vi "ge_PreviewWfm.vi"(6 "Rate Class":T1, 7 "ChassisCfg":refnum<class "ChassisCfg.lvclass">, 8 "error in":errorcluster, 10 "Chassis Name":string, 11 "Selected Group":refnum<class "ChanGrp.lvclass">) -> (0 "error out":errorcluster)   [LabVIEW 2012]
uses:
  Classes/Cfg Grandmaster/Class Chan Group/ChanGrp.lvclass
  Classes/Cfg Grandmaster/Class Chassis Cfg/ChassisCfg.lvclass
  Common/Controls/TE_Designator.ctl
  <vilib>/Utility/miscctls.llb/LVRowAndColumnTypeDef.ctl
  Classes/Cfg Grandmaster/Class Chan Group/Read GroupChans.vi
  Classes/Cfg Grandmaster/Class Chan Group/Read GrpName.vi
  Classes/Cfg Grandmaster/Class Chan Group/Read MeasType.vi
  Classes/Cfg Grandmaster/Class Timing Group/Read Rate.vi
  Classes/Measurements/Class Channel/Read ChanName.vi
  Classes/Measurements/Class Channel/Read Alias.vi
  Classes/Measurements/Class Channel/Channel.lvclass
  Classes/Cfg Grandmaster/Class Timing Group/TimingGrp.lvclass
panel:
  in  "Legend LB":i32[](listbox)
  out "Wfm Graph":waveform(sgl)[](graph)
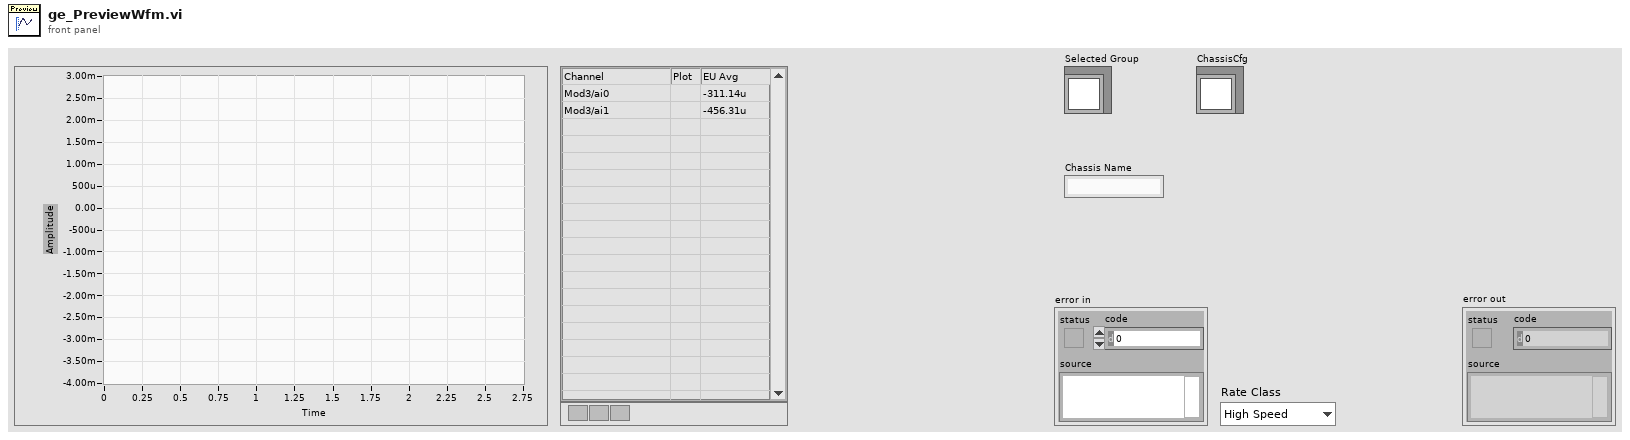
[diagram p1: front panel]
types:
  T1 = typedef "TE_Designator.ctl" = enum16{"High Speed", "Low Speed"}
  T2 = typedef "ge_MeasType.ctl" = enum16{"Voltage", "Frequency", "Tachometer", "Dynamic", "Thermocouple", "RTD", "Strain", "Current", "Resistance"}
  T3 = typedef "LVRowAndColumnTypeDef.ctl" = cluster{"Row":i32, "Column":i32}
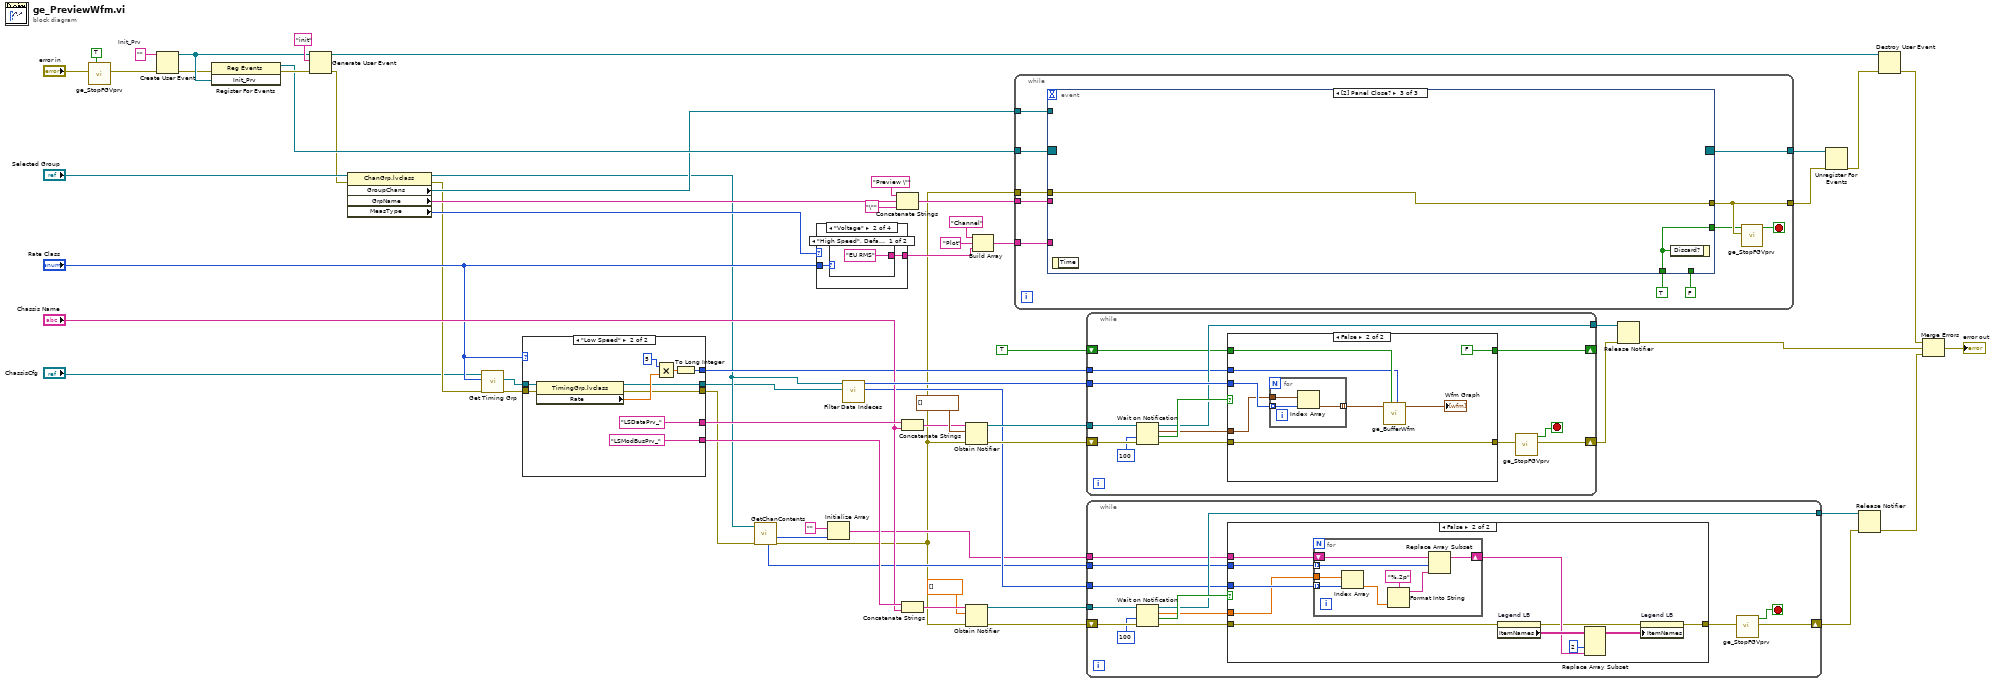
[diagram p0: block diagram]
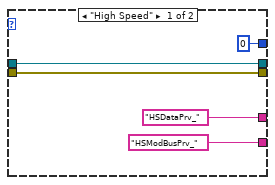
[diagram p2: hidden frame]
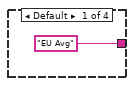
[diagram p3: hidden frame]
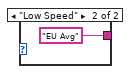
[diagram p4: hidden frame]
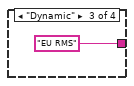
[diagram p5: hidden frame]
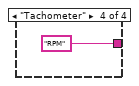
[diagram p6: hidden frame]
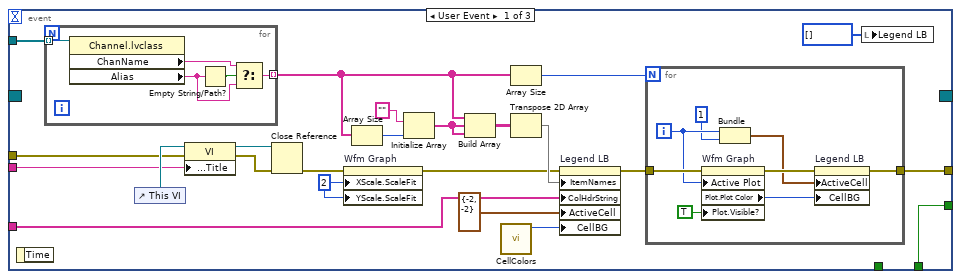
[diagram p8: hidden frame]
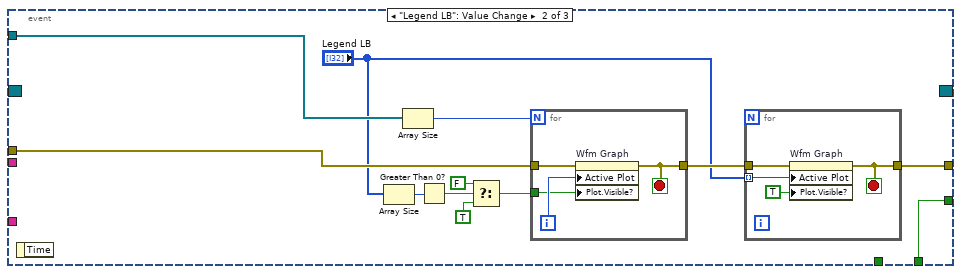
[diagram p9: hidden frame]
diagram:
  w60 = ""  # Init_Prv
  n1 = call "ge_StopFGVprv.vi"("Reset (F)"=TRUE, "error in"="error in") -> ("error out"=w11:errorcluster)  [unwired: 8 in, 1 out]
  n2 = Create User Event(user event datatype=w60, error in=w11) -> (user event=w58:refnum<user-event>, error out=w57:errorcluster)
  n3 = register-events(error in=w57, w58) -> (reference out=w56:refnum<event-registration>, error out=w59:errorcluster)  [unwired: 1 in]
  n4 = Generate User Event(user event=w58, event data cluster="init" ("event data"), error in=w59) -> (user event out=w54:refnum<user-event>, error out=w10:errorcluster)
  n5 = property class="ChanGrp.lvclass"(reference="Selected Group", error in=w10) -> (reference out=w2:refnum<class "ChanGrp.lvclass">, error out=w5:errorcluster, "GroupChans"=w12:refnum<class "Channel.lvclass">[], "GrpName"=w15:string, "MeasType"=w14:T2)
  n6 = call "Get Timing Grp.vi"("error in (no error)"=w5, "Timing Engine"="Rate Class", "Chassis Cfg"="ChassisCfg") -> ("error out"=w4:errorcluster, "Timing Groups"=w6:refnum<class "TimingGrp.lvclass">)  [unwired: 6 in, 1 out]
  n7 = case shown="\"Low Speed\"" "Rate Class" {
    tunnel: ["HSDataPrv_" ("name (unnamed)") "LSDataPrv_" ("name (unnamed)")] -> w42
    tunnel: ["HSModBusPrv_" ("name (unnamed)") "LSModBusPrv_" ("name (unnamed)")] -> w36
    tunnel: [w63 w70] -> w1
    tunnel: [0 w72] -> w16
    tunnel: w6 -> [w63 w69]
    tunnel: w4 -> [w62 w68]
    tunnel: [w62 w67] -> w9
    frame "High Speed" {
    }
    frame "Low Speed" {
      n8 = property class="TimingGrp.lvclass"(reference=w69, error in=w68) -> (reference out=w70:refnum<class "TimingGrp.lvclass">, error out=w67:errorcluster, "Rate"=w71:dbl)
      n9 = Multiply(x=5, y=w71) -> (x*y=w73:dbl)
      n10 = To Long Integer(number=w73) -> (32bit integer=w72:i32)
    }
  }
  n11 = call "GetChanContents.vi"("error in"=w9, "ChanGrp.lvclass"=w2) -> ("error out"=w8:errorcluster, "Num of Chans"=w25:i32, "Chans w/ Modbus"=w22:i32[])  [unwired: 3 in, 4 out]
  n12 = case shown="\"Voltage\"" w14 {
    tunnel: ["EU Avg" w79 "EU RMS" "RPM"] -> w19
    tunnel: "Rate Class" -> [_ w78 _ _]
    frame Default {
    }
    frame "Voltage" {
      n13 = case shown="\"High Speed\", Default" w78 {
        tunnel: ["EU RMS" "EU Avg"] -> w79
        frame "High Speed", Default {
        }
        frame "Low Speed" {
        }
      }
    }
    frame "Dynamic" {
    }
    frame "Tachometer" {
    }
  }
  n14 = Initialize Array("", w25) -> (w23:string[])
  n15 = call "Filter Data Indeces.vi"("TimingGrp.lvclass"=w1, "Selected Group"=w2) -> ("MB Chan Indeces"=w26:i32[], "Selected Chan Indeces"=w37:i32[])  [unwired: 7 in, 1 out]
  n16 = Concatenate Strings("Preview \"", w15, "\"") -> (w40:string)
  n17 = Concatenate Strings(w42, "Chassis Name") -> (w41:string)
  n18 = Concatenate Strings(w36, "Chassis Name") -> (w34:string)
  n19 = Obtain Notifier(name (unnamed)=w41, notification data type=waveform(sgl)[] [] ("data"), error in (no error)=w8) -> (notifier out=w47:refnum<notifier>, error out=w33:errorcluster)  [unwired: 1 in, 1 out]
  n20 = Obtain Notifier(name (unnamed)=w34, notification data type=dbl[] [], error in (no error)=w8) -> (notifier out=w30:refnum<notifier>, error out=w31:errorcluster)  [unwired: 1 in, 1 out]
  n21 = Build Array("Channel", "Plot", w19) -> (w18:string[])
  n22 = while {
    tunnel: w8 -> [w93]
    tunnel: w56 -> [w92]
    tunnel: [w91] -> w53
    tunnel: [w89] -> w52
    tunnel: w12 -> [w86]
    tunnel: w40 -> [w85]
    tunnel: w18 -> [w84]
    stop <- w87 stop-if-true
    n23 = event shown="[2] Panel Close?" {
      selector: w92 -> [_ _ _]
      dyn-events: [_ _ _] -> w91
      timeout: _ -> [_ _ _]
      tunnel: TRUE ("Discard?") -> [_ _ w152]
      tunnel: w93 -> [w102 w140 w151]
      tunnel: FALSE ("Discard?") -> [w114 w141 _]
      tunnel: [w112 w142 w151] -> w89
      tunnel: [w114 w141 w152] -> w88
      tunnel: w86 -> [w95 w137 _]
      tunnel: w85 -> [w101 _ _]
      tunnel: w84 -> [w96 _ _]
      event User Event {
        w108 = u8 2 ("X Scale.Scale Fit")
        n24 = event-data() -> ()  [unwired: 1 in, 1 out]
        n25 = for {
          tunnel: [w121] -> w100 mode=indexing
          tunnel: w95 -> [w118] mode=indexing
          n26 = property class="Channel.lvclass"(reference=w118) -> ("ChanName"=w119:string, "Alias"=w120:string)  [unwired: 1 in, 2 out]
          n27 = Empty String/Path?(string/path=w120) -> (empty?=w122:bool)
          n28 = Select(t=w119, s=w122, f=w120) -> (s? t:f=w121:string)
        }
        n29 = control-ref of="This VI"() -> (w104:refnum<vi>)
        n30 = property class="VI"(reference=w104, error in=w102, "Front Panel.Title"=w101) -> (reference out=w105:refnum<vi>, error out=w106:errorcluster)
        n31 = Close Reference(reference=w105, error in (no error)=w106) -> (error out=w103:errorcluster)
        n32 = property on="Wfm Graph" class="WFGraph (strict)"(error in=w103, "XScale.ScaleFit"=w108, "YScale.ScaleFit"=w108) -> (error out=w107:errorcluster)  [unwired: 1 in, 1 out]
        n33 = Array Size(array=w100) -> (size(s)=w115:i32)
        n34 = Initialize Array("", w115) -> (w98:string[])
        n35 = Build Array(w100, w98, w98) -> (w99:string[][])
        n36 = call "CellColors.vi"() -> ("Normal"=w113:u32)  [unwired: 8 in, 3 out]
        n37 = Array Size(array=w100) -> (size(s)=w110:i32)
        n38 = Transpose 2D Array(2D array=w99) -> (transposed array=w117:string[][])
        n39 = property on="Legend LB" class="MCListbox (strict)"(error in=w107, "ItemNames"=w117, "ColHdrString"=w96, "ActiveCell"=T3 {"Row"=-2, "Column"=-2} ("Active Cell:Active Cell"), "CellBG"=w113) -> (error out=w111:errorcluster)  [unwired: 1 in, 1 out]
        n40 = for {
          N: w110 -> [_]
          tunnel: [w130] -> w112
          tunnel: w111 -> [w128]
          i -> [w126]
          n41 = property on="Wfm Graph" class="WFGraph (strict)"(error in=w128, "Active Plot"=w126, "Plot.Visible?"=TRUE ("Plot.Visible")) -> (error out=w129:errorcluster, "Plot.Plot Color"=w127:u32)  [unwired: 1 in, 1 out]
          n42 = Bundle(w126, 1) -> (w124:cluster{i32, i32})  [unwired: 1 in]
          n43 = property on="Legend LB" class="MCListbox (strict)"(error in=w129, "ActiveCell"=w124, "CellBG"=w127) -> (error out=w130:errorcluster)  [unwired: 1 in, 1 out]
        }
        n44 = local write "Legend LB"(i32[] [] ("Legend LB")) -> ()
      }
      event "Legend LB": Value Change {
        n45 = event-data() -> ()  [unwired: 1 in, 1 out]
        n46 = Array Size(array="Legend LB") -> (size(s)=w135:i32)
        n47 = Array Size(array=w137) -> (size(s)=w138:i32)
        n48 = Greater Than 0?(x=w135) -> (x > 0?=w134:bool)
        n49 = Select(t=FALSE ("Plot.Visible"), s=w134, f=TRUE ("Plot.Visible")) -> (s? t:f=w131:bool)
        n50 = for {
          N: w138 -> [_]
          tunnel: w140 -> [w146]
          tunnel: [w145] -> w139
          tunnel: w131 -> [w143]
          i -> [w144]
          stop <- w145 stop-if-true
          n51 = property on="Wfm Graph" class="WFGraph (strict)"(error in=w146, "Active Plot"=w144, "Plot.Visible?"=w143) -> (error out=w145:errorcluster)  [unwired: 1 in, 1 out]
        }
        n52 = for {
          tunnel: w139 -> [w150]
          tunnel: [w147] -> w142
          tunnel: "Legend LB" -> [w149] mode=indexing
          stop <- w147 stop-if-true
          n53 = property on="Wfm Graph" class="WFGraph (strict)"(error in=w150, "Active Plot"=w149, "Plot.Visible?"=TRUE ("Plot.Visible")) -> (error out=w147:errorcluster)  [unwired: 1 in, 1 out]
        }
      }
      event Panel Close? {
        n54 = event-data() -> ()  [unwired: 1 in, 1 out]
        n55 = event-data("Discard?"=w152) -> ()  [unwired: 1 in, 1 out]
      }
    }
    n56 = call "ge_StopFGVprv.vi"("error in"=w89, "User stop? (F)"=w88) -> ("Stop?"=w87:bool)  [unwired: 8 in, 1 out]
  }
  n57 = while {
    shift-right: [w166] -> w45
    shift-left: w33 -> [w161]
    tunnel: w37 -> [w163]
    tunnel: w47 -> [w162]
    tunnel: [w156] -> w46
    shift-right: [w154] -> _
    shift-left: TRUE -> [w155]
    tunnel: w16 -> [w153]
    stop <- w164 stop-if-true
    n58 = Wait on Notification(notifier=w162, timeout in ms (-1)=100, error in (no error)=w161) -> (notifier out=w156:refnum<notifier>, notification=w158:waveform(sgl)[], timed out?=w159:bool, error out=w160:errorcluster)  [unwired: 1 in]
    n59 = case shown="False" w159 {
      tunnel: w160 -> [w168 w176]
      tunnel: [w168 w176] -> w165
      tunnel: w163 -> [_ w175]
      tunnel: w158 -> [_ w174]
      tunnel: w155 -> [w167 w171]
      tunnel: [w167 FALSE] -> w154
      tunnel: w153 -> [_ w169]
      frame True {
      }
      frame False {
        n60 = for {
          tunnel: w175 -> [w179] mode=indexing
          tunnel: w174 -> [w178]
          tunnel: [w177] -> w173 mode=indexing
          n61 = Index Array(array=w178, index=w179) -> (element=w177:waveform(sgl))
        }
        n62 = call "ge_BufferWfm.vi"("Wfm In"=w173, "Reset?"=w171, "Chart History"=w169) -> ("Wfm Out"=→"Wfm Graph":waveform(sgl)[])  [unwired: 6 in]
      }
    }
    n63 = call "ge_StopFGVprv.vi"("error in"=w165) -> ("error out"=w166:errorcluster, "Stop?"=w164:bool)  [unwired: 9 in]
  }
  n64 = while {
    shift-right: [w192] -> w28
    shift-left: w31 -> [w188]
    tunnel: w30 -> [w189]
    tunnel: [w183] -> w29
    tunnel: w26 -> [w182]
    tunnel: w23 -> [w181]
    tunnel: w22 -> [w180]
    stop <- w190 stop-if-true
    n65 = Wait on Notification(notifier=w189, timeout in ms (-1)=100, error in (no error)=w188) -> (notifier out=w183:refnum<notifier>, notification=w185:dbl[], timed out?=w186:bool, error out=w187:errorcluster)  [unwired: 1 in]
    n66 = case shown="False" w186 {
      tunnel: w187 -> [w193 w201]
      tunnel: [w193 w195] -> w191
      tunnel: w185 -> [_ w203]
      tunnel: w182 -> [_ w204]
      tunnel: w181 -> [_ w202]
      tunnel: w180 -> [_ w194]
      frame True {
      }
      frame False {
        n67 = for {
          tunnel: w204 -> [w212] mode=indexing
          tunnel: w203 -> [w211]
          shift-right: [w209] -> w199
          shift-left: w202 -> [w210]
          tunnel: w194 -> [w208] mode=indexing
          n68 = Index Array(array=w211, index=w212) -> (element=w206:dbl)
          n69 = Format Into String(format string="%.2p", w206) -> (resulting string=w205:string)  [unwired: 2 in, 1 out]
          n70 = Replace Array Subset(array=w210, new element=w205, index=w208) -> (w209:string[])
        }
        n71 = property on="Legend LB" class="MCListbox (strict)"(error in=w201) -> (error out=w197:errorcluster, "ItemNames"=w200:string[][])  [unwired: 1 in, 1 out]
        n72 = Replace Array Subset(array=w200, new element=w199, index (col)=2 ("disabled index (col)")) -> (w196:string[][])  [unwired: 1 in]
        n73 = property on="Legend LB" class="MCListbox (strict)"(error in=w197, "ItemNames"=w196) -> (error out=w195:errorcluster)  [unwired: 1 in, 1 out]
      }
    }
    n74 = call "ge_StopFGVprv.vi"("error in"=w191) -> ("error out"=w192:errorcluster, "Stop?"=w190:bool)  [unwired: 9 in]
  }
  n75 = Release Notifier(notifier=w46, error in (no error)=w45) -> (error out=w44:errorcluster)  [unwired: 1 in, 2 out]
  n76 = Unregister For Events(event registration refnum=w53, error in=w52) -> (error out=w55:errorcluster)
  n77 = Release Notifier(notifier=w29, error in (no error)=w28) -> (error out=w27:errorcluster)  [unwired: 1 in, 2 out]
  n78 = Destroy User Event(user event=w54, error in=w55) -> (error out=w51:errorcluster)
  n79 = Merge Errors(w51, w44, w27) -> (→"error out":errorcluster)
